vi "Frac Decimation test.vi"() -> ()   [LabVIEW 2013]
uses:
  <vilib>/Platform/TimedLoop/XDataNode/timing_clust.ctl
  <vilib>/Platform/TimedLoop/XDataNode/nitl_modes.ctl
  <vilib>/Platform/TimedLoop/XDataNode/wakeup.ctl
  <vilib>/rvi/Emulation/niFpgaSctlEmulationGetInTimedLoop.vi
  <vilib>/rvi/Emulation/niFpgaEmulationReportErrorSimple.vi
  <vilib>/rvi/Emulation/niFpgaGetClockAttributes.vi
  <vilib>/rvi/Emulation/niFpgaCriticalErrorInLSC.vi
  <vilib>/rvi/IPIntegrationNode/IPINode_Utilities/niFpgaIPINodeSimCore.vi
  <vilib>/rvi/eio/common/nirviEmuTemplateMethod_errors.vi
  <vilib>/rvi/Emulation/niFpgaProcessEmulError.vi
  <vilib>/Platform/TimedLoop/XDataNode/XDataNode.xnode
  <vilib>/rvi/XilinxIP/XIPIN_XNode/niFpgaXIPIN.xnode
  Frac Decimation test/FIR Compiler/FractionalDecimationV1.dll
  <vilib>/rvi/IPIntegrationNode/IPINode_Xnode/niFpgaIPINode.xnode
  <vilib>/rvi/FXPMathLib/FxpInterpret/XNode/nifxpmath_Interpret.xnode
  <vilib>/eio/EIONode/EIONode.xnode
  <vilib>/Platform/TimedLoop/XDataNode/XDNodeRunTimeDep.lvlib
panel:
  out "rdy":bool
  out "AO":fxp<+/-,33,33>
  in  "IO Module\\AI 0":i16
  out "Element":i16
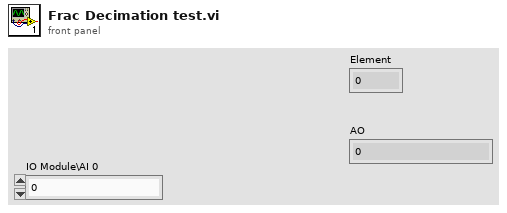
[diagram p1: front panel]
types:
  T1 = typedef "XDNodeRunTimeDep.lvlib/timing_clust.ctl" = cluster{"Expected End [f-1]":u64, "Actual End [f-1]":u64, "Finished Late? [f-1]":bool, "Expected End [i-1]":u64, "Actual End [i-1]":u64, "Finished Late? [i-1]":bool, "Expected Start [i]":u64, "Actual Start [i]":u64, "Expected Start [f]":u64, "Actual Start [f]":u64, "Source Name":string, "Structure Name":string, "Period":i64, "Deadline":i64, "Offset":i64, "Start":i64, "Priority":i32, "Timeout":i32, "Mode":T2, "Wakeup Reason":T3, "Error":errorcluster, "Source Type":string, "Secondary Source Type":string, "Global End Time":u64, "Global Start Time":u64, "Frame Duration":u64, "Iteration Duration":u64, "Assigned CPU":i32, "I/O Scan Engine Mode":u32}
  T2 = typedef "XDNodeRunTimeDep.lvlib/nitl_modes.ctl" = enum32{"No Change", "Process missed periods, maintain original phase", "Discard missed periods, maintain original phase", "Process missed periods, ignore original phase", "Discard missed periods, ignore original phase"}
  T3 = typedef "XDNodeRunTimeDep.lvlib/wakeup.ctl" = enum32{"Normal", "Aborted", "Asynchronous wakeup", "Timing source error", "Timed loop error", "Timeout"}
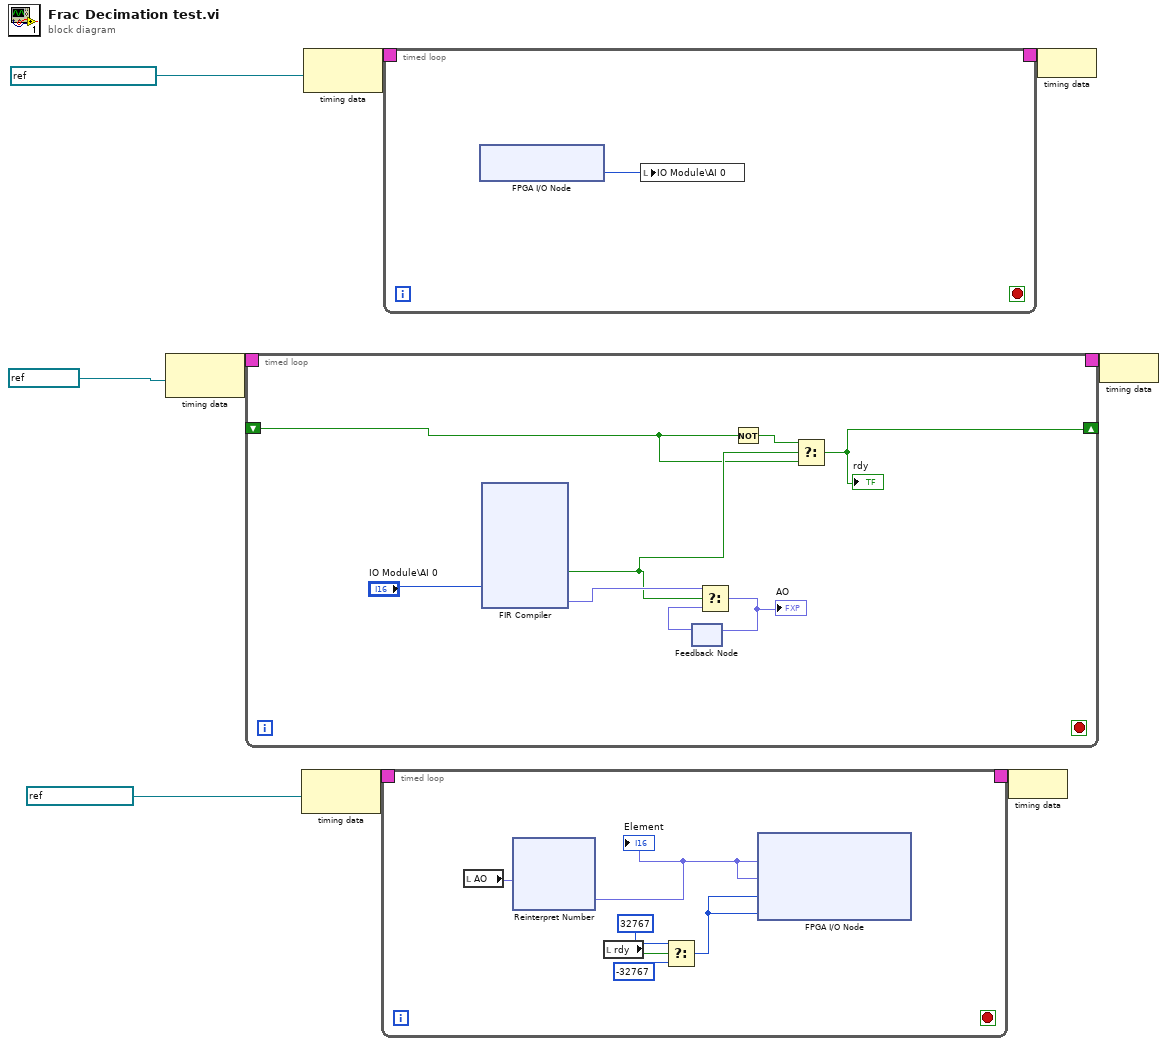
[diagram p0: block diagram]
diagram:
  n1 = node-c288(refnum<k21> "300MHz" ("Source Name")) -> (w9:T1)
  n2 = timed-loop {
    timing: w9 -> [_]
    timing-out: [_] -> w8
    shift-right: [w10] -> _
    shift-left: _ -> [w11]
    stop <- _ stop-if-true
    n3 = xnode ("FIR Compiler")("din"="IO Module\\AI 0") -> ("rdy"=w13:bool, "dout"=w17:fxp<+/-,33,33>)  [unwired: 1 out]
    n4 = feedback #1() -> (w15:fxp<+/-,33,33>)  [unwired: 1 in]
    n5 = Select(t=w17, s=w13, f=w15) -> (s? t:f=w16:fxp<+/-,33,33>)
    "AO" <- w16
    n6 = feedback-in #1(w16) -> ()
    n7 = Not(x=w11) -> (.not. x?=w12:bool)
    n8 = Select(t=w12, s=w13, f=w11) -> (s? t:f=w10:bool)
    "rdy" <- w10
  }
  n9 = node-c288(refnum<k21> "100 MHz Clock" ("Source Name")) -> (w6:T1)
  n10 = node-c288(refnum<k21> "IO Module\\Data Clock" ("Source Name")) -> (w3:T1)
  n11 = timed-loop {
    timing: w6 -> [_]
    timing-out: [_] -> w5
    stop <- _ stop-if-true
    n12 = local read "AO"() -> (w73:fxp<+/-,33,33>)
    n13 = xnode "Reinterpret Number"("x"=w73) -> ("y"=w72:fxp<+/-,33,16>)
    "Element" <- w72
    n14 = local read "rdy"() -> (w71:bool)
    n15 = Select(t=i16 32767 ("IO Module\\AO 1 N-1"), s=w71, f=i16 -32767 ("IO Module\\AO 1 N-1")) -> (s? t:f=w68:i16)
    n16 = xnode "FPGA I/O Node"("IO Module\\AO 0 N-1"=w72, "IO Module\\AO 0 N"=w72, "IO Module\\AO 1 N-1"=w68, "IO Module\\AO 1 N"=w68) -> ()  [unwired: 4 in, 4 out]
  }
  n17 = timed-loop {
    timing: w3 -> [_]
    timing-out: [_] -> w2
    stop <- _ stop-if-true
    n18 = xnode "FPGA I/O Node"() -> ("IO Module\\AI 0"=w76:i16)  [unwired: 1 in, 1 out]
    n19 = local write "IO Module\\AI 0"(w76) -> ()
  }
  n20 = node-c288(w5) -> ()
  n21 = node-c288(w2) -> ()
  n22 = node-c288(w8) -> ()
